vi "NewUser.vi"(2 "error in (no error)":errorcluster, 3 "Byte Stream File in":refnum<file>) -> (0 "error out":errorcluster, 1 "Byte Stream File out":refnum<file>)   [LabVIEW 2017]
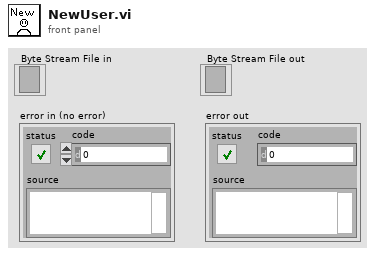
[diagram p1: front panel]
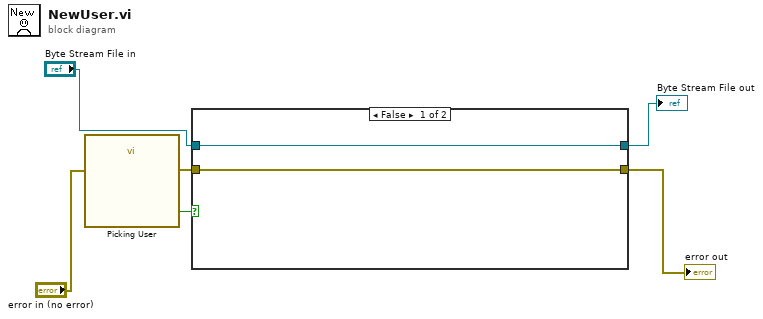
[diagram p0: block diagram]
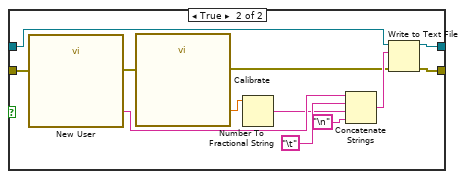
[diagram p2: hidden frame]
diagram:
  n1 = call "Picking User"("error in (no error)"="error in (no error)") -> ("New User?"=w1:bool, "error out"=w6:errorcluster)  [unwired: 16 in, 1 out]
  n2 = case shown="False" w1 {
    tunnel: w6 -> [w7 w11]
    tunnel: "Byte Stream File in" -> [w8 w14]
    tunnel: [w8 w13] -> w3
    tunnel: [w7 w12] -> w4
    frame False {
    }
    frame True {
      n3 = call "New User"("error in (no error)"=w11) -> ("New User Name"=w20:string, "error out"=w10:errorcluster)  [unwired: 16 in, 1 out]
      n4 = call "Calibrate"("error in (no error)"=w10) -> ("Calibration Value?"=w17:dbl, "error out"=w9:errorcluster)  [unwired: 16 in, 1 out]
      n5 = Number To Fractional String(number=w17) -> (F-format string=w16:string)  [unwired: 3 in]
      n6 = Concatenate Strings(w20, "\t", w16, "\n" ("string")) -> (w19:string)
      n7 = Write to Text File(file (use dialog)=w14, text=w19, error in=w9) -> (refnum out=w13:refnum<file>, error out=w12:errorcluster)  [unwired: 1 in, 1 out]
    }
  }
  "error out" <- w4
  "Byte Stream File out" <- w3
